vi "Set Enablel.vi"(8 "error in (no error)":errorcluster, 10 "Enable?":bool, 11 "Handle in":i32) -> (0 "error out":errorcluster, 3 "Handle out":i32)   [LabVIEW 2013, in "Thorlabs_MC2000B.lvlib"]
uses:
  <instrlib>/Thorlabs_MC2000B/Thorlabs_MC2000B.lvlib
  Program Files/National Instruments/LabVIEW 2011/instr.lib/Thorlabs_MC2000B/Library/MC2000CommandLibWin64.dll
  <instrlib>/Thorlabs_MC2000B/Library/MC2000CommandLibWin32.dll
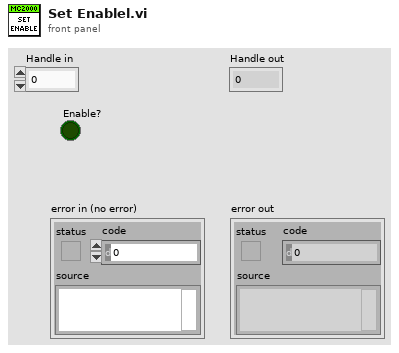
[diagram p1: front panel]
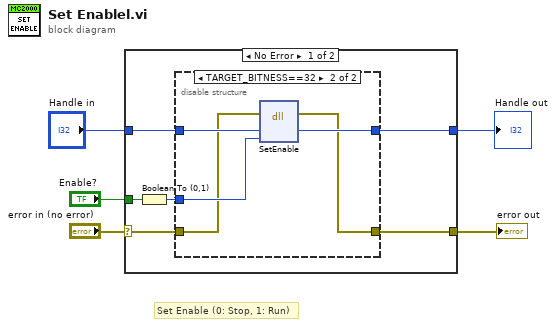
[diagram p0: block diagram]
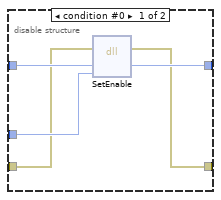
[diagram p2: hidden frame]
diagram:
  # "Set Enable (0: Stop, 1: Run)"
  n1 = case shown="No Error" "error in (no error)" {
    selector: "error in (no error)" -> [w6 w23]
    tunnel: [w7 w23] -> w5
    tunnel: "Enable?" -> [w11 _]
    tunnel: "Handle in" -> [w9 w22]
    tunnel: [w8 w22] -> w1
    frame No Error {
      n2 = Boolean To (0,1)(Boolean=w11) -> (0, 1=w10:i16)
      n3 = disable-structure shown="TARGET_BITNESS==32" {
        disable-tunnel: w10 -> [w16 w21]
        disable-tunnel: w9 -> [w15 w20]
        disable-tunnel: [w14 w19] -> w8
        disable-tunnel: [w13 w18] -> w7
        disable-tunnel: w6 -> [w12 w17]
        frame condition #0 {
          n4 = dll-call lib="D:/Program Files/National Instruments/LabVIEW 2011/instr.lib/Thorlabs_MC2000B/Library/MC2000CommandLibWin64.dll" fn="SetEnable"(error in=w12, "hdl"=w15, "enable"=w16) -> (error out=w13:errorcluster, "hdl"=w14:i32)  [unwired: 4 in, 1 out]
        }
        frame condition #1 (active) {
          n5 = dll-call lib="C:/Program Files (x86)/National Instruments/LabVIEW 2013/instr.lib/Thorlabs_MC2000B/Library/MC2000CommandLibWin32.dll" fn="SetEnable"(error in=w17, "hdl"=w20, "enable"=w21) -> (error out=w18:errorcluster, "hdl"=w19:i32)  [unwired: 4 in, 1 out]
        }
      }
    }
    frame Error {
    }
  }
  "error out" <- w5
  "Handle out" <- w1
